vi "dequeueMessage.vi"(8 "error in (no error)":errorcluster) -> (0 "error out":errorcluster, 3 "message out":T1)   [LabVIEW 2017, in "loggingModule.lvlib"]
uses:
  loggingModule.lvlib
  TypeDefs/message.ctl
  TypeDefs/queueFGVState.ctl
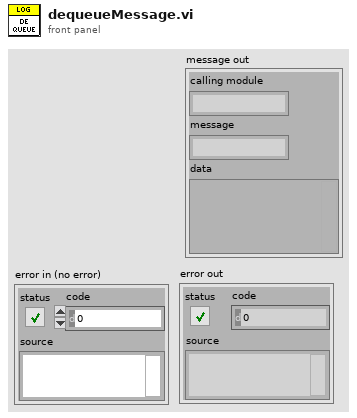
[diagram p1: front panel]
types:
  T1 = typedef "loggingModule.lvlib/message.ctl" = cluster{"calling module":string, "message":string, "data":variant}
  T2 = typedef "loggingModule.lvlib/queueFGVState.ctl" = enum16{"set", "get"}
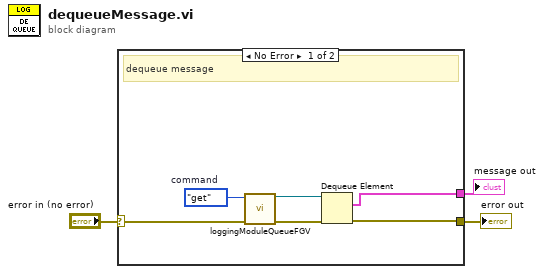
[diagram p0: block diagram]
diagram:
  n1 = case shown="No Error" "error in (no error)" {
    selector: "error in (no error)" -> [w9 w10]
    tunnel: [w7 w10] -> w2
    tunnel: [w5 _] -> w1
    frame No Error {
      w4 = queueFGVState."get"  # command
      # "dequeue message"
      n2 = call "loggingModuleQueueFGV.vi"("error in (no error)"=w9, "command"=w4) -> ("error out"=w8:errorcluster, "queue out"=w6:refnum<queue>)  [unwired: 8 in]
      n3 = Dequeue Element(queue=w6, error in (no error)=w8) -> (element=w5:T1, error out=w7:errorcluster)  [unwired: 1 in, 2 out]
    }
    frame Error {
    }
  }
  "error out" <- w2
  "message out" <- w1
